vi "Map MiniGUIs.vi"(8 "error in (no error)":errorcluster, 9 "MiniGUI":refnum<class "Message Enqueuer.lvclass">, 10 "key":string, 11 "LabGUI in":refnum<class "LabGUI.lvclass">) -> (0 "error out":errorcluster, 3 "LabGUI out":refnum<class "LabGUI.lvclass">)   [LabVIEW 2019, in "LabGUI.lvlib" / "LabGUI.lvclass"]
uses:
  LabGUI.lvclass
  <vilib>/ActorFramework/Message Enqueuer/Message Enqueuer.lvclass
  LabGUI.lvclass/LabGUI.ctl
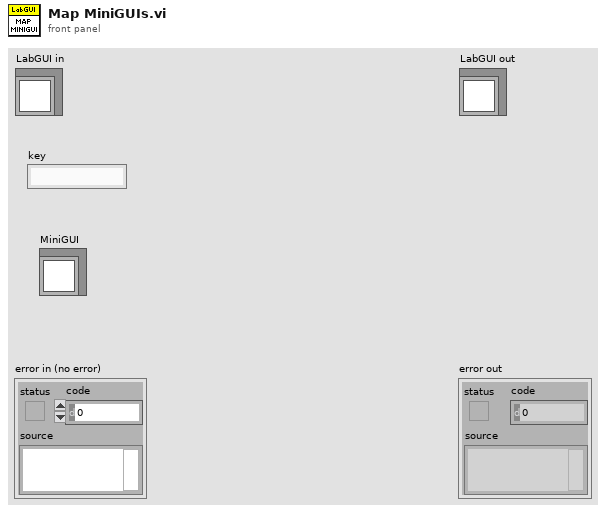
[diagram p1: front panel]
types:
  T1 = map{string, refnum<class "Message Enqueuer.lvclass">}
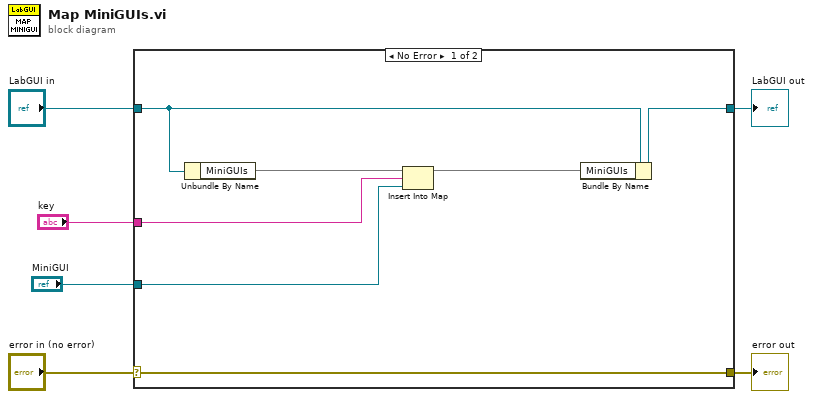
[diagram p0: block diagram]
diagram:
  n1 = case shown="No Error" "error in (no error)" {
    selector: "error in (no error)" -> [w13 w15]
    tunnel: [w13 w15] -> w5
    tunnel: [w9 w14] -> w3
    tunnel: "LabGUI in" -> [w10 w14]
    tunnel: "key" -> [w11 _]
    tunnel: "MiniGUI" -> [w7 _]
    frame No Error {
      n2 = Unbundle By Name(w10) -> ("MiniGUIs"=w12:T1)
      n3 = Insert Into Map(map in=w12, key=w11, value=w7) -> (map out=w8:T1)  [unwired: 2 out]
      n4 = Bundle By Name(cluster=w10, "MiniGUIs"=w8) -> (w9:refnum<class "LabGUI.lvclass">)
    }
    frame Error {
    }
  }
  "error out" <- w5
  "LabGUI out" <- w3
